vi "CheckHeaderCode.vi"(8 "error in":errorcluster, 10 "Code":string, 11 "Headers":string="HTTP/1.1 200 OK\r\nServer: nginx/1.17.6\r\nDate: Thu, 04 Nov 2021 12:06:49 GMT\r\nContent-Type: application/json\r\nContent-Length: 12191\r\nConnection: keep-alive\r\nVary: Accept-Encoding\r\nVary: Accept, Accept-Encoding, Accept-Language, Cookie\r\nAllow: GET, POST, HEAD, OPTIONS\r\nX-Frame-Options: DENY\r\nContent-Language: it\r\nX-Content-Type-Options: nosniff\r\nX-XSS-Protection: 1; mode=block\r\nCache-Control: no-cache=\"Set-Cookie\"\r\n\r\n") -> (0 "error out":errorcluster)   [LabVIEW 2019, in "ByteGSWebAPI.lvlib" / "ByteGSWebAPI-V0.lvclass"]
doc: "Cerca un determinato codice nella prima riga di Header, se non trova restituisce un errore \"BadResponse\""
uses:
  ByteGSWebAPI-V0.lvclass
  <vilib>/regexp/Match Regular Expression.xnode
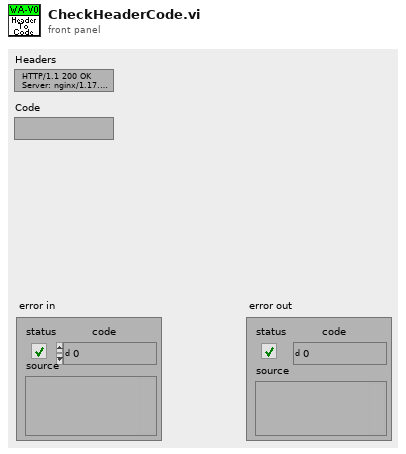
[diagram p1: front panel]
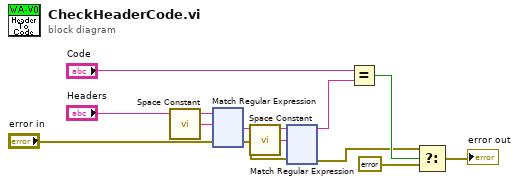
[diagram p0: block diagram]
diagram:
  n1 = call <vilib>:"Space Constant.vi"() -> ("String"=w10:string)
  n2 = xnode "Match Regular Expression"("input string"="Headers", "regular expression"=w10, "error in"="error in") -> ("after match"=w11:string, "error out"=w7:errorcluster)  [unwired: 3 in, 3 out]
  n3 = call <vilib>:"Space Constant.vi"() -> ("String"=w9:string)
  n4 = xnode "Match Regular Expression"("input string"=w11, "regular expression"=w9, "error in"=w7) -> ("before match"=w5:string, "error out"=w2:errorcluster)  [unwired: 3 in, 3 out]
  n5 = Equal?(x="Code", y=w5) -> (x = y?=w4:bool)
  n6 = Select(t=w2, s=w4, f=errorcluster {"status"=TRUE, "code"=0, "source"="BadResponse"} ("error out")) -> (s? t:f=→"error out":errorcluster)
